vi "ma_SML RBW.vi"(1 "RBW definition":enum16{"3dB", "6dB", "ENBW", "bin width"}(ring), 2 "window":u16(ring) items=["Rectangle"=0, "Hanning"=1, "Hamming"=2, "Blackman-Harris"=3, "Exact Blackman"=4, "Blackman"=5, "Flat Top"=6, "4 Term B-Harris "=7, "7 Term B-Harris"=8, "Low Sidelobe"=9, "Blackman Nuttall"=11, "Triangle"=30, "Bartlett-Hanning"=31, "Bohman"=32, "Parzen"=33, "Welch"=34, "Kaiser"=60, "Dolph-Chebyshev"=61, "Gaussian"=62], 3 "window size":i32=-1, 4 "fs":dbl format="%.2f") -> (0 "RBW":dbl format="%.2f")   [LabVIEW 2020, in "NI_MAPro.lvlib"]
uses:
  NI_MAPro.lvlib
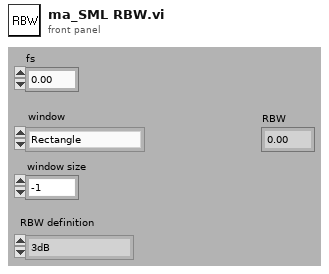
[diagram p1: front panel]
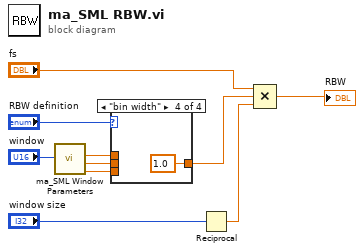
[diagram p0: block diagram]
diagram:
  n1 = call "ma_SML Window Parameters.vi"("window"="window") -> ("ENBW"=w4:dbl, "3dB BW"=w3:dbl, "6dB BW"=w2:dbl)  [unwired: 1 out]
  n2 = case shown="\"bin width\"" "RBW definition" {
    tunnel: w4 -> [_ _ w13 _]
    tunnel: w3 -> [w11 _ _ _]
    tunnel: w2 -> [_ w12 _ _]
    tunnel: [w11 w12 w13 1.0 ("ENBW")] -> w1
    frame "3dB", Default {
    }
    frame "6dB" {
    }
    frame "ENBW" {
    }
    frame "bin width" {
    }
  }
  n3 = Reciprocal(x="window size") -> (1/x=w8:dbl)
  n4 = Compound Arithmetic op=MULTIPLY("fs", w1, w8) -> (→"RBW":dbl)
